vi "Show Live Data on XY Graph with Buffer LV2012 NI Verified.vi"() -> ()   [LabVIEW 2012]
panel:
  out "XY Graph":cluster{dbl[], dbl[]}(graph)
  in  "Buffer Size(Points)":i32=1000
  in  "Milliseconds to wait":u32=200
  in  "stop":bool
  # "Overview: This VI shows a technique to display live data on XY Line Graph with a memory buffer \nRequirements: LabVIEW 2012 (or compatible)\nInstructions:\n1. Run the VI"
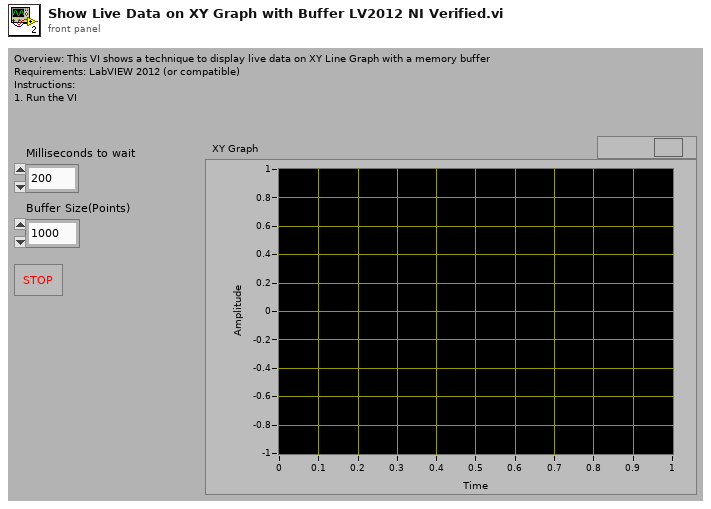
[diagram p1: front panel]
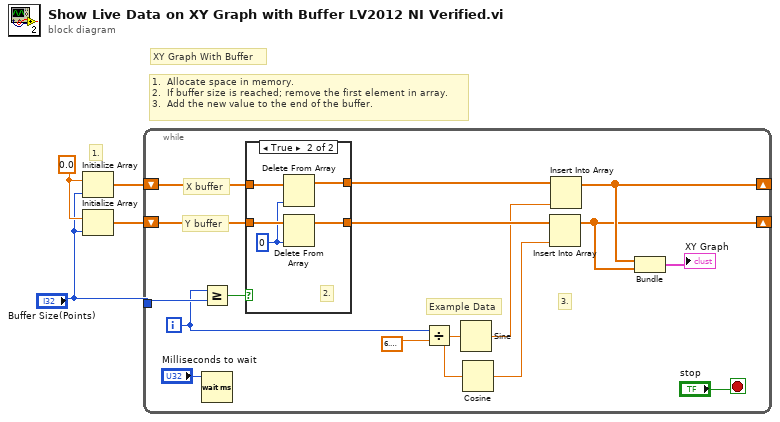
[diagram p0: block diagram]
diagram:
  w2 = 0.0
  # "XY Graph With Buffer"
  # "1.  Allocate space in memory.\n2.  If buffer size is reached; remove the first element in array.\n3.  Add the new value to the end of the buffer."
  # "1."
  n1 = Initialize Array(w2, "Buffer Size(Points)") -> (w4:dbl[])
  n2 = Initialize Array(w2, "Buffer Size(Points)") -> (w3:dbl[])
  n3 = while {
    shift-right: [w9] -> _
    shift-left: w4 -> [w19]
    shift-right: [w8] -> _
    shift-left: w3 -> [w17]
    tunnel: "Buffer Size(Points)" -> [w13]
    i -> [w6]
    stop <- "stop" stop-if-true
    # "Example Data"
    # "3."
    # "Y buffer"
    # "X buffer"
    n4 = Greater Or Equal?(x=w6, y=w13) -> (x >= y?=w15:bool)
    n5 = Wait (ms)(milliseconds to wait="Milliseconds to wait") -> ()  [unwired: 1 out]
    n6 = case shown="True" w15 {
      tunnel: w19 -> [w22 w27]
      tunnel: [w22 w26] -> w18
      tunnel: w17 -> [w21 w25]
      tunnel: [w21 w24] -> w16
      frame False {
      }
      frame True {
        w23 = 0 ("index")
        # "2."
        n7 = Delete From Array(array=w27, index=w23) -> (array with subset deleted=w26:dbl[])  [unwired: 1 in, 1 out]
        n8 = Delete From Array(array=w25, index=w23) -> (array with subset deleted=w24:dbl[])  [unwired: 1 in, 1 out]
      }
    }
    n9 = Divide(x=w6, y=6.283185307179586) -> (x/y=w10:dbl)
    n10 = Sine(x=w10) -> (sin(x)=w12:dbl)
    n11 = Cosine(x=w10) -> (cos(x)=w11:dbl)
    n12 = Insert Into Array(array=w16, new element=w11) -> (w8:dbl[])  [unwired: 1 in]
    n13 = Insert Into Array(array=w18, new element=w12) -> (w9:dbl[])  [unwired: 1 in]
    n14 = Bundle(w9, w8) -> (→"XY Graph":cluster{dbl[], dbl[]})  [unwired: 1 in]
  }
